vi "movethetatest.vi"() -> ()   [LabVIEW 2018]
panel:
  out "ThetaOut (rad)":dbl
  in  "Theta":dbl
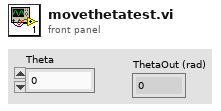
[diagram p1: front panel]
types:
  T1 = enum16{"Standard", "Buffered", "CRLF", "Immediate"}
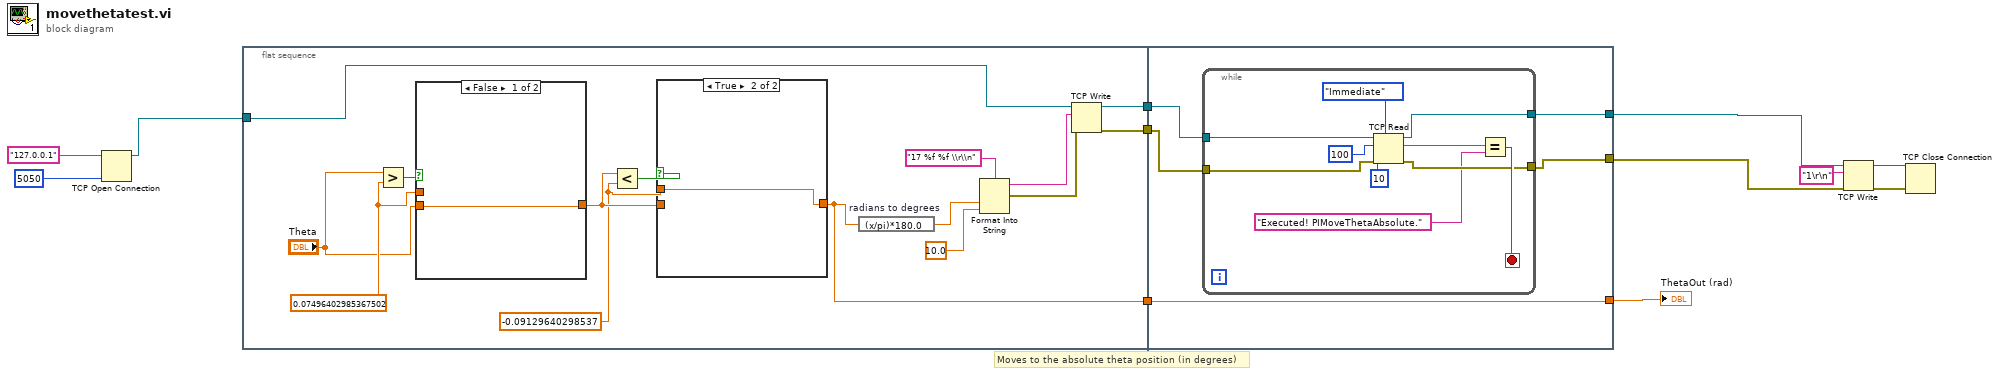
[diagram p0: block diagram]
diagram:
  # "Moves to the absolute theta position (in degrees)"
  n1 = TCP Open Connection(address="127.0.0.1", remote port or service name=u16 5050) -> (connection ID=w6:refnum<k5>)  [unwired: 3 in, 1 out]
  n2 = flat-sequence {
    tunnel: [w25] -> w12
    tunnel: [w24] -> w11
    tunnel: w6 -> [w17]
    tunnel: [w14] -> w10
    tunnel: w12 -> [w35]
    tunnel: w11 -> [w36]
    tunnel: [w34] -> w2
    tunnel: [w33] -> w1
    tunnel: [w32] -> w9
    tunnel: w10 -> [w32]
    frame #0 {
      w19 = 0.07496402985367502 ("y")
      w18 = -0.09129640298537 ("y")
      n3 = Greater?(x="Theta", y=w19) -> (0:w21:bool)
      n4 = case shown="False" w21 {
        tunnel: "Theta" -> [w30 _]
        tunnel: [w30 w31] -> w20
        tunnel: w19 -> [_ w31]
        frame False {
        }
        frame True {
        }
      }
      n5 = Less?(x=w20, y=w18) -> (x < y?=w23:bool)
      n6 = case shown="True" w23 {
        tunnel: [w28 w29] -> w14
        tunnel: w20 -> [w28 _]
        tunnel: w18 -> [_ w29]
        frame False {
        }
        frame True {
        }
      }
      n7 = expression code="(x/pi)*180.0" "radians to degrees"(w14) -> (w13:dbl)
      n8 = Format Into String(format string="17 %f %f \\r\\n", w13, 10.0 ("input 3")) -> (resulting string=w26:string, error out=w27:errorcluster)  [unwired: 2 in]
      n9 = TCP Write(connection ID=w17, data in=w26, error in (no error)=w27) -> (connection ID out=w25:refnum<k5>, error out=w24:errorcluster)  [unwired: 1 in, 1 out]
    }
    frame #1 {
      n10 = while {
        tunnel: w36 -> [w44]
        tunnel: [w40] -> w33
        tunnel: [w39] -> w34
        tunnel: w35 -> [w37]
        stop <- w41 stop-if-true
        n11 = TCP Read(connection ID=w37, bytes to read=100, error in (no error)=w44, 7:T1."Immediate" ("mode (standard)"), 9:10 ("timeout ms (25000)")) -> (connection ID out=w39:refnum<k5>, data out=w42:string, error out=w40:errorcluster)
        n12 = Equal?(x=w42, y="Executed! PIMoveThetaAbsolute.") -> (x = y?=w41:bool)
      }
    }
  }
  n13 = TCP Write(connection ID=w2, data in="1\r\n", error in (no error)=w1) -> (connection ID out=w4:refnum<k5>, error out=w5:errorcluster)  [unwired: 1 in, 1 out]
  n14 = TCP Close Connection(connection ID=w4, error in (no error)=w5) -> ()  [unwired: 1 in, 2 out]
  "ThetaOut (rad)" <- w9
